vi "nanocal -- nuclear schottky fit V8.vi"() -> ()   [LabVIEW 2021] (continued)
\"στN\" -> 0.000000000000   ,  \"τ11 \" -> 0.000000000000   ,  \"τ12\" -> 0.000000000000   ,  \"τ22\" -> 0.000000000000   ,  \"τN1\" -> 0.000000000000   ,  \"τN2\" -> 0.000000000000   ,  \"σηlogτ1 \" -> 0.000000000000   ,  \"σηlogτS\" -> 0.000000000000   ,  \"σηlogτN\" -> 0.000000000000   ,  \"σlogτ1\" -> 0.000000000000   ,  \"σlogτS\" -> 0.000000000000   ,  \"σlogτN\" -> 0.000000000000   ,  \"σητ1\" -> 0.000000000000   ,  \"σητS \" -> 0.000000000000   ,  \"σητN\" -> 0.000000000000    |>   , \r\"IDS0648_220613_RAW_cal__ref_\" ->   <|    \"ζ\" -> 0.044166566928   ,  \"τ1\" -> 0.016574003526   ,  \"τS\" -> 0.032211448360   ,  \"τN\" -> 0.000936709307   ,  \"τC\" -> 0.001862438862   ,  \"κ0\" -> 0.000000003065   ,  \"mm1\" -> 0.000074801958   ,  \"mm2\" -> 0.015787727605   ,  \"mm3\" -> 0.037186110817   ,  \"T\" -> 0.520000000000   ,  \"B\" -> 6.000000000000   ,  \"θ\" -> 90.000000000000   ,  \"Reoff\" -> 0.000000000000   ,  \"Imoff\" -> 0.000000000000   ,  \"στ1\" -> 0.000113368552   ,  \"στS\" -> 0.000002764404   ,  \"στN\" -> 0.000003162403   ,  \"τ11 \" -> 0.000000000000   ,  \"τ12\" -> 0.000000000000   ,  \"τ22\" -> 0.000000000000   ,  \"τN1\" -> 0.000000000000   ,  \"τN2\" -> 0.000000000000   ,  \"σηlogτ1 \" -> 0.169044191232   ,  \"σηlogτS\" -> 0.000346748172   ,  \"σηlogτN\" -> 0.139725969375   ,  \"σlogτ1\" -> 0.006840142890   ,  \"σlogτS\" -> 0.000085820552   ,  \"σlogτN\" -> 0.003376077471   ,  \"σητ1\" -> 0.002801739022   ,  \"σητS \" -> 0.000011169261   ,  \"σητN\" -> 0.000130882616    |>   , \r\"IDS0648_220613_RAW_cal__sam_\" ->   <|    \"ζ\" -> 0.000000000000   ,  \"τ1\" -> 0.000000000000   ,  \"τS\" -> 0.000000000000   ,  \"τN\" -> 0.000000000000   ,  \"τC\" -> 0.000000000000   ,  \"κ0\" -> 0.000000000000   ,  \"mm1\" -> 0.000000000000   ,  \"mm2\" -> 0.000000000000   ,  \"mm3\" -> 0.000000000000   ,  \"T\" -> 0.520000000000   ,  \"B\" -> 6.000000000000   ,  \"θ\" -> 90.000000000000   ,  \"Reoff\" -> 0.000000000000   ,  \"Imoff\" -> 0.000000000000   ,  \"στ1\" -> 0.000000000000   ,  \"στS\" -> 0.000000000000   ,  \"στN\" -> 0.000000000000   ,  \"τ11 \" -> 0.000000000000   ,  \"τ12\" -> 0.000000000000   ,  \"τ22\" -> 0.000000000000   ,  \"τN1\" -> 0.000000000000   ,  \"τN2\" -> 0.000000000000   ,  \"σηlogτ1 \" -> 0.000000000000   ,  \"σηlogτS\" -> 0.000000000000   ,  \"σηlogτN\" -> 0.000000000000   ,  \"σlogτ1\" -> 0.000000000000   ,  \"σlogτS\" -> 0.000000000000   ,  \"σlogτN\" -> 0.000000000000   ,  \"σητ1\" -> 0.000000000000   ,  \"σητS \" -> 0.000000000000   ,  \"σητN\" -> 0.000000000000    |>   , \r\"IDS0649_220613_RAW_cal__ref_\" ->   <|    \"ζ\" -> 0.036098260006   ,  \"τ1\" -> 0.019839922246   ,  \"τS\" -> 0.028557133674   ,  \"τN\" -> 0.000530751010   ,  \"τC\" -> 0.002125743780   ,  \"κ0\" -> 0.000000003752   ,  \"mm1\" -> 0.000069248734   ,  \"mm2\" -> 0.019012462839   ,  \"mm3\" -> 0.033021861161   ,  \"T\" -> 0.620000000000   ,  \"B\" -> 6.000000000000   ,  \"θ\" -> 90.000000000000   ,  \"Reoff\" -> 0.000000000000   ,  \"Imoff\" -> 0.000000000000   ,  \"στ1\" -> 0.000292189890   ,  \"στS\" -> 0.000002960548   ,  \"στN\" -> 0.000003977957   ,  \"τ11 \" -> 0.000000000000   ,  \"τ12\" -> 0.000000000000   ,  \"τ22\" -> 0.000000000000   ,  \"τN1\" -> 0.000000000000   ,  \"τN2\" -> 0.000000000000   ,  \"σηlogτ1 \" -> 0.142367105799   ,  \"σηlogτS\" -> 0.000145255254   ,  \"σηlogτN\" -> 0.135095367098   ,  \"σlogτ1\" -> 0.014727370701   ,  \"σlogτS\" -> 0.000103671054   ,  \"σlogτN\" -> 0.007494959556   ,  \"σητ1\" -> 0.002824552309   ,  \"σητS \" -> 0.000004148074   ,  \"σητN\" -> 0.000071702003    |>   , \r\"IDS0649_220613_RAW_cal__sam_\" ->   <|    \"ζ\" -> 0.000000000000   ,  \"τ1\" -> 0.000000000000   ,  \"τS\" -> 0.000000000000   ,  \"τN\" -> 0.000000000000   ,  \"τC\" -> 0.000000000000   ,  \"κ0\" -> 0.000000000000   ,  \"mm1\" -> 0.000000000000   ,  \"mm2\" -> 0.000000000000   ,  \"mm3\" -> 0.000000000000   ,  \"T\" -> 0.620000000000   ,  \"B\" -> 6.000000000000   ,  \"θ\" -> 90.000000000000   ,  \"Reoff\" -> 0.000000000000   ,  \"Imoff\" -> 0.000000000000   ,  \"στ1\" -> 0.000000000000   ,  \"στS\" -> 0.000000000000   ,  \"στN\" -> 0.000000000000   ,  \"τ11 \" -> 0.000000000000   ,  \"τ12\" -> 0.000000000000   ,  \"τ22\" -> 0.000000000000   ,  \"τN1\" -> 0.000000000000   ,  \"τN2\" -> 0.000000000000   ,  \"σηlogτ1 \" -> 0.000000000000   ,  \"σηlogτS\" -> 0.000000000000   ,  \"σηlogτN\" -> 0.000000000000   ,  \"σlogτ1\" -> 0.000000000000   ,  \"σlogτS\" -> 0.000000000000   ,  \"σlogτN\" -> 0.000000000000   ,  \"σητ1\" -> 0.000000000000   ,  \"σητS \" -> 0.000000000000   ,  \"σητN\" -> 0.000000000000    |>   , \r\"IDS0650_220613_RAW_cal__ref_\" ->   <|    \"ζ\" -> 0.026767413186   ,  \"τ1\" -> 0.019958900137   ,  \"τS\" -> 0.023153953288   ,  \"τN\" -> 0.000189088054   ,  \"τC\" -> 0.002398350564   ,  \"κ0\" -> 0.000000005121   ,  \"mm1\" -> 0.000056918136   ,  \"mm2\" -> 0.019398352629   ,  \"mm3\" -> 0.026869854111   ,  \"T\" -> 0.820000000000   ,  \"B\" -> 6.000000000000   ,  \"θ\" -> 90.000000000000   ,  \"Reoff\" -> 0.000000000000   ,  \"Imoff\" -> 0.000000000000   ,  \"στ1\" -> 0.000637008577   ,  \"στS\" -> 0.000002061875   ,  \"στN\" -> 0.000003206406   ,  \"τ11 \" -> 0.000000000000   ,  \"τ12\" -> 0.000000000000   ,  \"τ22\" -> 0.000000000000   ,  \"τN1\" -> 0.000000000000   ,  \"τN2\" -> 0.000000000000   ,  \"σηlogτ1 \" -> 0.127380236705   ,  \"σηlogτS\" -> 0.000047088453   ,  \"σηlogτN\" -> 0.132172067620   ,  \"σlogτ1\" -> 0.031916016057   ,  \"σlogτS\" -> 0.000089050669   ,  \"σlogτN\" -> 0.016957208977   ,  \"σητ1\" -> 0.002542369424   ,  \"σητS \" -> 0.000001090284   ,  \"σητN\" -> 0.000024992159    |>   , \r\"IDS0650_220613_RAW_cal__sam_\" ->   <|    \"ζ\" -> 0.000000000000   ,  \"τ1\" -> 0.000000000000   ,  \"τS\" -> 0.000000000000   ,  \"τN\" -> 0.000000000000   ,  \"τC\" -> 0.000000000000   ,  \"κ0\" -> 0.000000000000   ,  \"mm1\" -> 0.000000000000   ,  \"mm2\" -> 0.000000000000   ,  \"mm3\" -> 0.000000000000   ,  \"T\" -> 0.820000000000   ,  \"B\" -> 6.000000000000   ,  \"θ\" -> 90.000000000000   ,  \"Reoff\" -> 0.000000000000   ,  \"Imoff\" -> 0.000000000000   ,  \"στ1\" -> 0.000000000000   ,  \"στS\" -> 0.000000000000   ,  \"στN\" -> 0.000000000000   ,  \"τ11 \" -> 0.000000000000   ,  \"τ12\" -> 0.000000000000   ,  \"τ22\" -> 0.000000000000   ,  \"τN1\" -> 0.000000000000   ,  \"τN2\" -> 0.000000000000   ,  \"σηlogτ1 \" -> 0.000000000000   ,  \"σηlogτS\" -> 0.000000000000   ,  \"σηlogτN\" -> 0.000000000000   ,  \"σlogτ1\" -> 0.000000000000   ,  \"σlogτS\" -> 0.000000000000   ,  \"σlogτN\" -> 0.000000000000   ,  \"σητ1\" -> 0.000000000000   ,  \"σητS \" -> 0.000000000000   ,  \"σητN\" -> 0.000000000000    |>   , \r\"IDS0651_220613_RAW_cal__ref_\" ->   <|    \"ζ\" -> 0.024620092111   ,  \"τ1\" -> 0.015537036119   ,  \"τS\" -> 0.019312906027   ,  \"τN\" -> 0.000067030104   ,  \"τC\" -> 0.002705916622   ,  \"κ0\" -> 0.000000007154   ,  \"mm1\" -> 0.000057343864   ,  \"mm2\" -> 0.015387205435   ,  \"mm3\" -> 0.022655475386   ,  \"T\" -> 1.120000000000   ,  \"B\" -> 6.000000000000   ,  \"θ\" -> 90.000000000000   ,  \"Reoff\" -> 0.000000000000   ,  \"Imoff\" -> 0.000000000000   ,  \"στ1\" -> 0.001880910040   ,  \"στS\" -> 0.000002935864   ,  \"στN\" -> 0.000004201788   ,  \"τ11 \" -> 0.000000000000   ,  \"τ12\" -> 0.000000000000   ,  \"τ22\" -> 0.000000000000   ,  \"τN1\" -> 0.000000000000   ,  \"τN2\" -> 0.000000000000   ,  \"σηlogτ1 \" -> 0.134633854477   ,  \"σηlogτS\" -> 0.000023496461   ,  \"σηlogτN\" -> 0.133516099454   ,  \"σlogτ1\" -> 0.121059771335   ,  \"σlogτS\" -> 0.000152015645   ,  \"σlogτN\" -> 0.062685083512   ,  \"σητ1\" -> 0.002091811060   ,  \"σητS \" -> 0.000000453785   ,  \"σητN\" -> 0.000008949598    |>   , \r\"IDS0651_220613_RAW_cal__sam_\" ->   <|    \"ζ\" -> 0.000000000000   ,  \"τ1\" -> 0.000000000000   ,  \"τS\" -> 0.000000000000   ,  \"τN\" -> 0.000000000000   ,  \"τC\" -> 0.000000000000   ,  \"κ0\" -> 0.000000000000   ,  \"mm1\" -> 0.000000000000   ,  \"mm2\" -> 0.000000000000   ,  \"mm3\" -> 0.000000000000   ,  \"T\" -> 1.120000000000   ,  \"B\" -> 6.000000000000   ,  \"θ\" -> 90.000000000000   ,  \"Reoff\" -> 0.000000000000   ,  \"Imoff\" -> 0.000000000000   ,  \"στ1\" -> 0.000000000000   ,  \"στS\" -> 0.000000000000   ,  \"στN\" -> 0.000000000000   ,  \"τ11 \" -> 0.000000000000   ,  \"τ12\" -> 0.000000000000   ,  \"τ22\" -> 0.000000000000   ,  \"τN1\" -> 0.000000000000   ,  \"τN2\" -> 0.000000000000   ,  \"σηlogτ1 \" -> 0.000000000000   ,  \"σηlogτS\" -> 0.000000000000   ,  \"σηlogτN\" -> 0.000000000000   ,  \"σlogτ1\" -> 0.000000000000   ,  \"σlogτS\" -> 0.000000000000   ,  \"σlogτN\" -> 0.000000000000   ,  \"σητ1\" -> 0.000000000000   ,  \"σητS \" -> 0.000000000000   ,  \"σητN\" -> 0.000000000000    |>   , \r\"IDS0652_220613_RAW_cal__ref_\" ->   <|    \"ζ\" -> 0.018133168210   ,  \"τ1\" -> 0.015564889407   ,  \"τS\" -> 0.014281099211   ,  \"τN\" -> 0.000013869214   ,  \"τC\" -> 0.003052925154   ,  \"κ0\" -> 0.000000012545   ,  \"mm1\" -> 0.000045053166   ,  \"mm2\" -> 0.015460375194   ,  \"mm3\" -> 0.017666567693   ,  \"T\" -> 1.900000000000   ,  \"B\" -> 6.000000000000   ,  \"θ\" -> 90.000000000000   ,  \"Reoff\" -> 0.000000000000   ,  \"Imoff\" -> 0.000000000000   ,  \"στ1\" -> 0.007531531497   ,  \"στS\" -> 0.000002103829   ,  \"στN\" -> 0.000003717358   ,  \"τ11 \" -> 0.000000000000   ,  \"τ12\" -> 0.000000000000   ,  \"τ22\" -> 0.000000000000   ,  \"τN1\" -> 0.000000000000   ,  \"τN2\" -> 0.000000000000   ,  \"σηlogτ1 \" -> 0.117619771927   ,  \"σηlogτS\" -> 0.000004424081   ,  \"σηlogτN\" -> 0.130136475948   ,  \"σlogτ1\" -> 0.483879538125   ,  \"σlogτS\" -> 0.000147315653   ,  \"σlogτN\" -> 0.268029442413   ,  \"σητ1\" -> 0.001830738742   ,  \"σητS \" -> 0.000000063181   ,  \"σητN\" -> 0.000001804891    |>   , \r\"IDS0652_220613_RAW_cal__sam_\" ->   <|    \"ζ\" -> 0.000000000000   ,  \"τ1\" -> 0.000000000000   ,  \"τS\" -> 0.000000000000   ,  \"τN\" -> 0.000000000000   ,  \"τC\" -> 0.000000000000   ,  \"κ0\" -> 0.000000000000   ,  \"mm1\" -> 0.000000000000   ,  \"mm2\" -> 0.000000000000   ,  \"mm3\" -> 0.000000000000   ,  \"T\" -> 1.900000000000   ,  \"B\" -> 6.000000000000   ,  \"θ\" -> 90.000000000000   ,  \"Reoff\" -> 0.000000000000   ,  \"Imoff\" -> 0.000000000000   ,  \"στ1\" -> 0.000000000000   ,  \"στS\" -> 0.000000000000   ,  \"στN\" -> 0.000000000000   ,  \"τ11 \" -> 0.000000000000   ,  \"τ12\" -> 0.000000000000   ,  \"τ22\" -> 0.000000000000   ,  \"τN1\" -> 0.000000000000   ,  \"τN2\" -> 0.000000000000   ,  \"σηlogτ1 \" -> 0.000000000000   ,  \"σηlogτS\" -> 0.000000000000   ,  \"σηlogτN\" -> 0.000000000000   ,  \"σlogτ1\" -> 0.000000000000   ,  \"σlogτS\" -> 0.000000000000   ,  \"σlogτN\" -> 0.000000000000   ,  \"σητ1\" -> 0.000000000000   ,  \"σητS \" -> 0.000000000000   ,  \"σητN\" -> 0.000000000000    |>   , \r\"IDS0653_220613_RAW_cal__ref_\" ->   <|    \"ζ\" -> 0.015908509188   ,  \"τ1\" -> 0.015560123784   ,  \"τS\" -> 0.010437245612   ,  \"τN\" -> 0.000002583564   ,  \"τC\" -> 0.002705916622   ,  \"κ0\" -> 0.000000022391   ,  \"mm1\" -> 0.000033844139   ,  \"mm2\" -> 0.013260236096   ,  \"mm3\" -> 0.015577871465   ,  \"T\" -> 3.100000000000   ,  \"B\" -> 6.000000000000   ,  \"θ\" -> 90.000000000000   ,  \"Reoff\" -> 0.000000000000   ,  \"Imoff\" -> 0.000000000000   ,  \"στ1\" -> 0.028222346539   ,  \"στS\" -> 0.000001217229   ,  \"στN\" -> 0.000002849695   ,  \"τ11 \" -> 0.000000000000   ,  \"τ12\" -> 0.000000000000   ,  \"τ22\" -> 0.000000000000   ,  \"τN1\" -> 0.000000000000   ,  \"τN2\" -> 0.000000000000   ,  \"σηlogτ1 \" -> 0.102372166935   ,  \"σηlogτS\" -> 0.000000706034   ,  \"σηlogτN\" -> 0.126762129997   ,  \"σlogτ1\" -> 1.813761055527   ,  \"σlogτS\" -> 0.000116623590   ,  \"σlogτN\" -> 1.103009360706   ,  \"σητ1\" -> 0.001592923590   ,  \"σητS \" -> 0.000000007369   ,  \"σητN\" -> 0.000000327498    |>   , \r\"IDS0653_220613_RAW_cal__sam_\" ->   <|    \"ζ\" -> 0.000000000000   ,  \"τ1\" -> 0.000000000000   ,  \"τS\" -> 0.000000000000   ,  \"τN\" -> 0.000000000000   ,  \"τC\" -> 0.000000000000   ,  \"κ0\" -> 0.000000000000   ,  \"mm1\" -> 0.000000000000   ,  \"mm2\" -> 0.000000000000   ,  \"mm3\" -> 0.000000000000   ,  \"T\" -> 3.100000000000   ,  \"B\" -> 6.000000000000   ,  \"θ\" -> 90.000000000000   ,  \"Reoff\" -> 0.000000000000   ,  \"Imoff\" -> 0.000000000000   ,  \"στ1\" -> 0.000000000000   ,  \"στS\" -> 0.000000000000   ,  \"στN\" -> 0.000000000000   ,  \"τ11 \" -> 0.000000000000   ,  \"τ12\" -> 0.000000000000   ,  \"τ22\" -> 0.000000000000   ,  \"τN1\" -> 0.000000000000   ,  \"τN2\" -> 0.000000000000   ,  \"σηlogτ1 \" -> 0.000000000000   ,  \"σηlogτS\" -> 0.000000000000   ,  \"σηlogτN\" -> 0.000000000000   ,  \"σlogτ1\" -> 0.000000000000   ,  \"σlogτS\" -> 0.000000000000   ,  \"σlogτN\" -> 0.000000000000   ,  \"σητ1\" -> 0.000000000000   ,  \"σητS \" -> 0.000000000000   ,  \"σητN\" -> 0.000000000000    |>   , \r\"IDS0654_220613_RAW_cal__ref_\" ->   <|    \"ζ\" -> 0.019038104176   ,  \"τ1\" -> 0.015490030186   ,  \"τS\" -> 0.006638290269   ,  \"τN\" -> 0.000000433283   ,  \"τC\" -> 0.001884122649   ,  \"κ0\" -> 0.000000055099   ,  \"mm1\" -> 0.000027619939   ,  \"mm2\" -> 0.008620619838   ,  \"mm3\" -> 0.015491025321   ,  \"T\" -> 5.700000000000   ,  \"B\" -> 6.000000000000   ,  \"θ\" -> 90.000000000000   ,  \"Reoff\" -> 0.000000000000   ,  \"Imoff\" -> 0.000000000000   ,  \"στ1\" -> 0.134458541237   ,  \"στS\" -> 0.000000694139   ,  \"στN\" -> 0.000002640501   ,  \"τ11 \" -> 0.000000000000   ,  \"τ12\" -> 0.000000000000   ,  \"τ22\" -> 0.000000000000   ,  \"τN1\" -> 0.000000000000   ,  \"τN2\" -> 0.000000000000   ,  \"σηlogτ1 \" -> 0.085447105740   ,  \"σηlogτS\" -> 0.000000087953   ,  \"σηlogτN\" -> 0.122534708662   ,  \"σlogτ1\" -> 8.680327902656   ,  \"σlogτS\" -> 0.000104565901   ,  \"σlogτN\" -> 6.094171441911   ,  \"σητ1\" -> 0.001323578247   ,  \"σητS \" -> 0.000000000584   ,  \"σητN\" -> 0.000000053092    |>   , \r\"IDS0654_220613_RAW_cal__sam_\" ->   <|    \"ζ\" -> 0.000000000000   ,  \"τ1\" -> 0.000000000000   ,  \"τS\" -> 0.000000000000   ,  \"τN\" -> 0.000000000000   ,  \"τC\" -> 0.000000000000   ,  \"κ0\" -> 0.000000000000   ,  \"mm1\" -> 0.000000000000   ,  \"mm2\" -> 0.000000000000   ,  \"mm3\" -> 0.000000000000   ,  \"T\" -> 5.700000000000   ,  \"B\" -> 6.000000000000   ,  \"θ\" -> 90.000000000000   ,  \"Reoff\" -> 0.000000000000   ,  \"Imoff\" -> 0.000000000000   ,  \"στ1\" -> 0.000000000000   ,  \"στS\" -> 0.000000000000   ,  \"στN\" -> 0.000000000000   ,  \"τ11 \" -> 0.000000000000   ,  \"τ12\" -> 0.000000000000   ,  \"τ22\" -> 0.000000000000   ,  \"τN1\" -> 0.000000000000   ,  \"τN2\" -> 0.000000000000   ,  \"σηlogτ1 \" -> 0.000000000000   ,  \"σηlogτS\" -> 0.000000000000   ,  \"σηlogτN\" -> 0.000000000000   ,  \"σlogτ1\" -> 0.000000000000   ,  \"σlogτS\" -> 0.000000000000   ,  \"σlogτN\" -> 0.000000000000   ,  \"σητ1\" -> 0.000000000000   ,  \"σητS \" -> 0.000000000000   ,  \"σητN\" -> 0.000000000000    |>   , \r\"IDS0656_220614_RAW_cal__ref_\" ->   <|    \"ζ\" -> 0.110263031005   ,  \"τ1\" -> 0.036264946317   ,  \"τS\" -> 0.035363841561   ,  \"τN\" -> 0.002907549875   ,  \"τC\" -> 0.001147321567   ,  \"κ0\" -> 0.000000001565   ,  \"mm1\" -> 0.000111012610   ,  \"mm2\" -> 0.028483762527   ,  \"mm3\" -> 0.051308803803   ,  \"T\" -> 0.300000000000   ,  \"B\" -> 4.000000000000   ,  \"θ\" -> 90.000000000000   ,  \"Reoff\" -> 0.000000000000   ,  \"Imoff\" -> 0.000000000000   ,  \"στ1\" -> 0.000283051813   ,  \"στS\" -> 0.000006866298   ,  \"στN\" -> 0.000012798500   ,  \"τ11 \" -> 0.000000000000   ,  \"τ12\" -> 0.000000000000   ,  \"τ22\" -> 0.000000000000   ,  \"τN1\" -> 0.000000000000   ,  \"τN2\" -> 0.000000000000   ,  \"σηlogτ1 \" -> 0.116599052310   ,  \"σηlogτS\" -> 0.000355346389   ,  \"σηlogτN\" -> 0.130406494845   ,  \"σlogτ1\" -> 0.007805107735   ,  \"σlogτS\" -> 0.000194161553   ,  \"σlogτN\" -> 0.004401816116   ,  \"σητ1\" -> 0.004228458373   ,  \"σητS \" -> 0.000012566413   ,  \"σητN\" -> 0.000379163388    |>   , \r\"IDS0656_220614_RAW_cal__sam_\" ->   <|    \"ζ\" -> 0.000000000000   ,  \"τ1\" -> 0.000000000000   ,  \"τS\" -> 0.000000000000   ,  \"τN\" -> 0.000000000000   ,  \"τC\" -> 0.000000000000   ,  \"κ0\" -> 0.000000000000   ,  \"mm1\" -> 0.000000000000   ,  \"mm2\" -> 0.000000000000   ,  \"mm3\" -> 0.000000000000   ,  \"T\" -> 0.300000000000   ,  \"B\" -> 4.000000000000   ,  \"θ\" -> 90.000000000000   ,  \"Reoff\" -> 0.000000000000   ,  \"Imoff\" -> 0.000000000000   ,  \"στ1\" -> 0.000000000000   ,  \"στS\" -> 0.000000000000   ,  \"στN\" -> 0.000000000000   ,  \"τ11 \" -> 0.000000000000   ,  \"τ12\" -> 0.000000000000   ,  \"τ22\" -> 0.000000000000   ,  \"τN1\" -> 0.000000000000   ,  \"τN2\" -> 0.000000000000   ,  \"σηlogτ1 \" -> 0.000000000000   ,  \"σηlogτS\" -> 0.000000000000   ,  \"σηlogτN\" -> 0.000000000000   ,  \"σlogτ1\" -> 0.000000000000   ,  \"σlogτS\" -> 0.000000000000   ,  \"σlogτN\" -> 0.000000000000   ,  \"σητ1\" -> 0.000000000000   ,  \"σητS \" -> 0.000000000000   ,  \"σητN\" -> 0.000000000000    |>   , \r"
  in  "string IN":string="  \"IDS0158_210310_RAW_cal__ref_\" ->   <|    \"ζ\" -> 0.342934102355   ,  \"τ1\" -> 0.037912336866   ,  \"τS\" -> 0.322770587290   ,  \"τN\" -> 0.224517468406   ,  \"τC\" -> 0.000970428995   ,  \"κ0\" -> 0.000000000517   ,  \"mm1\" -> 0.000247395955   ,  \"mm2\" -> 0.021898106728   ,  \"mm3\" -> 0.751709056984   ,  \"T\" -> 0.120000000000   ,  \"B\" -> 12.000000000000   ,  \"θ\" -> 0.000000000000   ,  \"Reoff\" -> 0.000000000000   ,  \"Imoff\" -> 0.000000000000   ,  \"στ1\" -> 0.000893425914   ,  \"στS\" -> 0.002489408176   ,  \"στN\" -> 0.002611842121   ,  \"τ11 \" -> 0.000000000000   ,  \"τ12\" -> 0.000000000000   ,  \"τ22\" -> 0.000000000000   ,  \"τN1\" -> 0.000000000000   ,  \"τN2\" -> 0.000000000000   ,  \"σηlogτ1 \" -> 0.114569772809   ,  \"σηlogτS\" -> 0.007573309274   ,  \"σηlogτN\" -> 0.068166495911   ,  \"σlogτ1\" -> 0.023565572257   ,  \"σlogτS\" -> 0.007712623993   ,  \"σlogτN\" -> 0.011633135451   ,  \"σητ1\" -> 0.004343607821   ,  \"σητS \" -> 0.002444441482   ,  \"σητN\" -> 0.015304569092    |>   , \n\"IDS0158_210310_RAW_cal__sam_\" ->   <|    \"ζ\" -> 0.286336668596   ,  \"τ1\" -> 0.037477267671   ,  \"τS\" -> 0.354459287884   ,  \"τN\" -> 0.444916383639   ,  \"τC\" -> 0.001225600579   ,  \"κ0\" -> 0.000000000596   ,  \"mm1\" -> 0.000272242393   ,  \"mm2\" -> 0.016302418461   ,  \"mm3\" -> 1.050394445660   ,  \"T\" -> 0.120000000000   ,  \"B\" -> 12.000000000000   ,  \"θ\" -> 0.000000000000   ,  \"Reoff\" -> 0.000000000000   ,  \"Imoff\" -> 0.000000000000   ,  \"στ1\" -> 0.000000000000   ,  \"στS\" -> 0.000000000000   ,  \"στN\" -> 0.000000000000   ,  \"τ11 \" -> 0.000000000000   ,  \"τ12\" -> 0.000000000000   ,  \"τ22\" -> 0.000000000000   ,  \"τN1\" -> 0.000000000000   ,  \"τN2\" -> 0.000000000000   ,  \"σηlogτ1 \" -> 0.000000000000   ,  \"σηlogτS\" -> 0.000000000000   ,  \"σηlogτN\" -> 0.000000000000   ,  \"σlogτ1\" -> 0.000000000000   ,  \"σlogτS\" -> 0.000000000000   ,  \"σlogτN\" -> 0.000000000000   ,  \"σητ1\" -> 0.000000000000   ,  \"σητS \" -> 0.000000000000   ,  \"σητN\" -> 0.000000000000    |>   , \n\"IDS0159_210310_RAW_cal__ref_\" ->   <|    \"ζ\" -> 0.271761862806   ,  \"τ1\" -> 0.039955104592   ,  \"τS\" -> 0.227503722031   ,  \"τN\" -> 0.142080712192   ,  \"τC\" -> 0.000995450305   ,  \"κ0\" -> 0.000000000652   ,  \"mm1\" -> 0.000212140795   ,  \"mm2\" -> 0.023804196565   ,  \"mm3\" -> 0.486957606069   ,  \"T\" -> 0.150000000000   ,  \"B\" -> 12.000000000000   ,  \"θ\" -> 0.000000000000   ,  \"Reoff\" -> 0.000000000000   ,  \"Imoff\" -> 0.000000000000   ,  \"στ1\" -> 0.000698593116   ,  \"στS\" -> 0.001142949493   ,  \"στN\" -> 0.001230291496   ,  \"τ11 \" -> 0.000000000000   ,  \"τ12\" -> 0.000000000000   ,  \"τ22\" -> 0.000000000000   ,  \"τN1\" -> 0.000000000000   ,  \"τN2\" -> 0.000000000000   ,  \"σηlogτ1 \" -> 0.100498796621   ,  \"σηlogτS\" -> 0.005660617730   ,  \"σηlogτN\" -> 0.063140982058   ,  \"σlogτ1\" -> 0.017484452181   ,  \"σlogτS\" -> 0.005023871622   ,  \"σlogτN\" -> 0.008659102821   ,  \"σητ1\" -> 0.004015439930   ,  \"σητS \" -> 0.001287811603   ,  \"σητN\" -> 0.008971115699    |>   , \n\"IDS0159_210310_RAW_cal__sam_\" ->   <|    \"ζ\" -> 0.219100303741   ,  \"τ1\" -> 0.028643012604   ,  \"τS\" -> 0.279362928811   ,  \"τN\" -> 0.246156444058   ,  \"τC\" -> 0.001272401549   ,  \"κ0\" -> 0.000000000760   ,  \"mm1\" -> 0.000227975653   ,  \"mm2\" -> 0.014929571562   ,  \"mm3\" -> 0.655418694024   ,  \"T\" -> 0.150000000000   ,  \"B\" -> 12.000000000000   ,  \"θ\" -> 0.000000000000   ,  \"Reoff\" -> 0.000000000000   ,  \"Imoff\" -> 0.000000000000   ,  \"στ1\" -> 0.000000000000   ,  \"στS\" -> 0.000000000000   ,  \"στN\" -> 0.000000000000   ,  \"τ11 \" -> 0.000000000000   ,  \"τ12\" -> 0.000000000000   ,  \"τ22\" -> 0.000000000000   ,  \"τN1\" -> 0.000000000000   ,  \"τN2\" -> 0.000000000000   ,  \"σηlogτ1 \" -> 0.000000000000   ,  \"σηlogτS\" -> 0.000000000000   ,  \"σηlogτN\" -> 0.000000000000   ,  \"σlogτ1\" -> 0.000000000000   ,  \"σlogτS\" -> 0.000000000000   ,  \"σlogτN\" -> 0.000000000000   ,  \"σητ1\" -> 0.000000000000   ,  \"σητS \" -> 0.000000000000   ,  \"σητN\" -> 0.000000000000    |>   , \n\"IDS0160_210310_RAW_cal__ref_\" ->   <|    \"ζ\" -> 0.199613086212   ,  \"τ1\" -> 0.022193731398   ,  \"τS\" -> 0.116862561742   ,  \"τN\" -> 0.097247059130   ,  \"τC\" -> 0.001045881960   ,  \"κ0\" -> 0.000000000931   ,  \"mm1\" -> 0.000172948552   ,  \"mm2\" -> 0.011671612475   ,  \"mm3\" -> 0.268243755414   ,  \"T\" -> 0.180000000000   ,  \"B\" -> 12.000000000000   ,  \"θ\" -> 0.000000000000   ,  \"Reoff\" -> 0.000000000000   ,  \"Imoff\" -> 0.000000000000   ,  \"στ1\" -> 0.000089856815   ,  \"στS\" -> 0.000165029214   ,  \"στN\" -> 0.000188286128   ,  \"τ11 \" -> 0.000000000000   ,  \"τ12\" -> 0.000000000000   ,  \"τ22\" -> 0.000000000000   ,  \"τN1\" -> 0.000000000000   ,  \"τN2\" -> 0.000000000000   ,  \"σηlogτ1 \" -> 0.093550953866   ,  \"σηlogτS\" -> 0.006075230131   ,  \"σηlogτN\" -> 0.064015363974   ,  \"σlogτ1\" -> 0.004048747519   ,  \"σlogτS\" -> 0.001412164955   ,  \"σlogτN\" -> 0.001936162698   ,  \"σητ1\" -> 0.002076244742   ,  \"σητS \" -> 0.000709966956   ,  \"σητN\" -> 0.006225305886    |>   , \n\"IDS0160_210310_RAW_cal__sam_\" ->   <|    \"ζ\" -> 0.170488637524   ,  \"τ1\" -> 0.029234231120   ,  \"τS\" -> 0.149095458227   ,  \"τN\" -> 0.151792620275   ,  \"τC\" -> 0.001113424175   ,  \"κ0\" -> 0.000000001042   ,  \"mm1\" -> 0.000161291869   ,  \"mm2\" -> 0.013922632736   ,  \"mm3\" -> 0.368449807743   ,  \"T\" -> 0.180000000000   ,  \"B\" -> 12.000000000000   ,  \"θ\" -> 0.000000000000   ,  \"Reoff\" -> 0.000000000000   ,  \"Imoff\" -> 0.000000000000   ,  \"στ1\" -> 0.000000000000   ,  \"στS\" -> 0.000000000000   ,  \"στN\" -> 0.000000000000   ,  \"τ11 \" -> 0.000000000000   ,  \"τ12\" -> 0.000000000000   ,  \"τ22\" -> 0.000000000000   ,  \"τN1\" -> 0.000000000000   ,  \"τN2\" -> 0.000000000000   ,  \"σηlogτ1 \" -> 0.000000000000   ,  \"σηlogτS\" -> 0.000000000000   ,  \"σηlogτN\" -> 0.000000000000   ,  \"σlogτ1\" -> 0.000000000000   ,  \"σlogτS\" -> 0.000000000000   ,  \"σlogτN\" -> 0.000000000000   ,  \"σητ1\" -> 0.000000000000   ,  \"σητS \" -> 0.000000000000   ,  \"σητN\" -> 0.000000000000    |>   , \n\"IDS0161_210310_RAW_cal__ref_\" ->   <|    \"ζ\" -> 0.155485326727   ,  \"τ1\" -> 0.024589160211   ,  \"τS\" -> 0.103187251839   ,  \"τN\" -> 0.059327264902   ,  \"τC\" -> 0.001362397594   ,  \"κ0\" -> 0.000000001075   ,  \"mm1\" -> 0.000181522487   ,  \"mm2\" -> 0.014905594718   ,  \"mm3\" -> 0.198647580074   ,  \"T\" -> 0.200000000000   ,  \"B\" -> 12.000000000000   ,  \"θ\" -> 0.000000000000   ,  \"Reoff\" -> 0.000000000000   ,  \"Imoff\" -> 0.000000000000   ,  \"στ1\" -> 0.000106824093   ,  \"στS\" -> 0.000114207069   ,  \"στN\" -> 0.000127738509   ,  \"τ11 \" -> 0.000000000000   ,  \"τ12\" -> 0.000000000000   ,  \"τ22\" -> 0.000000000000   ,  \"τN1\" -> 0.000000000000   ,  \"τN2\" -> 0.000000000000   ,  \"σηlogτ1 \" -> 0.086294510505   ,  \"σηlogτS\" -> 0.004144737065   ,  \"σηlogτN\" -> 0.058529518145   ,  \"σlogτ1\" -> 0.004344357106   ,  \"σlogτS\" -> 0.001106794371   ,  \"σlogτN\" -> 0.002153116435   ,  \"σητ1\" -> 0.002121909544   ,  \"σητS \" -> 0.000427684027   ,  \"σητN\" -> 0.003472396228    |>   , \n\"IDS0161_210310_RAW_cal__sam_\" ->   <|    \"ζ\" -> 0.130531197151   ,  \"τ1\" -> 0.025704482770   ,  \"τS\" -> 0.129606657196   ,  \"τN\" -> 0.091602369165   ,  \"τC\" -> 0.001441379995   ,  \"κ0\" -> 0.000000001211   ,  \"mm1\" -> 0.000164978070   ,  \"mm2\" -> 0.014468182937   ,  \"mm3\" -> 0.262596407151   ,  \"T\" -> 0.200000000000   ,  \"B\" -> 12.000000000000   ,  \"θ\" -> 0.000000000000   ,  \"Reoff\" -> 0.000000000000   ,  \"Imoff\" -> 0.000000000000   ,  \"στ1\" -> 0.000000000000   ,  \"στS\" -> 0.000000000000   ,  \"στN\" -> 0.000000000000   ,  \"τ11 \" -> 0.000000000000   ,  \"τ12\" -> 0.000000000000   ,  \"τ22\" -> 0.000000000000   ,  \"τN1\" -> 0.000000000000   ,  \"τN2\" -> 0.000000000000   ,  \"σηlogτ1 \" -> 0.000000000000   ,  \"σηlogτS\" -> 0.000000000000   ,  \"σηlogτN\" -> 0.000000000000   ,  \"σlogτ1\" -> 0.000000000000   ,  \"σlogτS\" -> 0.000000000000   ,  \"σlogτN\" -> 0.000000000000   ,  \"σητ1\" -> 0.000000000000   ,  \"σητS \" -> 0.000000000000   ,  \"σητN\" -> 0.000000000000    |>   , \n\"IDS0162_210310_RAW_cal__ref_\" ->   <|    \"ζ\" -> 0.085932974943   ,  \"τ1\" -> 0.018822470857   ,  \"τS\" -> 0.068810147904   ,  \"τN\" -> 0.024216831887   ,  \"τC\" -> 0.001953952621   ,  \"κ0\" -> 0.000000001388   ,  \"mm1\" -> 0.000150968751   ,  \"mm2\" -> 0.013294741414   ,  \"mm3\" -> 0.108351778227   ,  \"T\" -> 0.250000000000   ,  \"B\" -> 12.000000000000   ,  \"θ\" -> 0.000000000000   ,  \"Reoff\" -> 0.000000000000   ,  \"Imoff\" -> 0.000000000000   ,  \"στ1\" -> 0.000058321163   ,  \"στS\" -> 0.000035049706   ,  \"στN\" -> 0.000037861271   ,  \"τ11 \" -> 0.000000000000   ,  \"τ12\" -> 0.000000000000   ,  \"τ22\" -> 0.000000000000   ,  \"τN1\" -> 0.000000000000   ,  \"τN2\" -> 0.000000000000   ,  \"σηlogτ1 \" -> 0.080513059924   ,  \"σηlogτS\" -> 0.002518022810   ,  \"σηlogτN\" -> 0.054257654253   ,  \"σlogτ1\" -> 0.003098486056   ,  \"σlogτS\" -> 0.000509368271   ,  \"σlogτN\" -> 0.001563427918   ,  \"σητ1\" -> 0.001515454724   ,  \"σητS \" -> 0.000173265522   ,  \"σητN\" -> 0.001313948492    |>   , \n\"IDS0162_210310_RAW_cal__sam_\" ->   <|    \"ζ\" -> 0.078258046754   ,  \"τ1\" -> 0.028009840731   ,  \"τS\" -> 0.092122038762   ,  \"τN\" -> 0.030129595899   ,  \"τC\" -> 0.001641062244   ,  \"κ0\" -> 0.000000001543   ,  \"mm1\" -> 0.000117303440   ,  \"mm2\" -> 0.019983073008   ,  \"mm3\" -> 0.141369335330   ,  \"T\" -> 0.250000000000   ,  \"B\" -> 12.000000000000   ,  \"θ\" -> 0.000000000000   ,  \"Reoff\" -> 0.000000000000   ,  \"Imoff\" -> 0.000000000000   ,  \"στ1\" -> 0.000000000000   ,  \"στS\" -> 0.000000000000   ,  \"στN\" -> 0.000000000000   ,  \"τ11 \" -> 0.000000000000   ,  \"τ12\" -> 0.000000000000   ,  \"τ22\" -> 0.000000000000   ,  \"τN1\" -> 0.000000000000   ,  \"τN2\" -> 0.000000000000   ,  \"σηlogτ1 \" -> 0.000000000000   ,  \"σηlogτS\" -> 0.000000000000   ,  \"σηlogτN\" -> 0.000000000000   ,  \"σlogτ1\" -> 0.000000000000   ,  \"σlogτS\" -> 0.000000000000   ,  \"σlogτN\" -> 0.000000000000   ,  \"σητ1\" -> 0.000000000000   ,  \"σητS \" -> 0.000000000000   ,  \"σητN\" -> 0.000000000000    |>   , \n\"IDS0163_210310_RAW_cal__ref_\" ->   <|    \"ζ\" -> 0.058825748663   ,  \"τ1\" -> 0.015012107932   ,  \"τS\" -> 0.052128918860   ,  \"τN\" -> 0.012953217864   ,  \"τC\" -> 0.002393557537   ,  \"κ0\" -> 0.000000001766   ,  \"mm1\" -> 0.000127725677   ,  \"mm2\" -> 0.011559700576   ,  \"mm3\" -> 0.074628881357   ,  \"T\" -> 0.300000000000   ,  \"B\" -> 12.000000000000   ,  \"θ\" -> 0.000000000000   ,  \"Reoff\" -> 0.000000000000   ,  \"Imoff\" -> 0.000000000000   ,  \"στ1\" -> 0.000023064935   ,  \"στS\" -> 0.000009573131   ,  \"στN\" -> 0.000010092664   ,  \"τ11 \" -> 0.000000000000   ,  \"τ12\" -> 0.000000000000   ,  \"τ22\" -> 0.000000000000   ,  \"τN1\" -> 0.000000000000   ,  \"τN2\" -> 0.000000000000   ,  \"σηlogτ1 \" -> 0.078709092172   ,  \"σηlogτS\" -> 0.001802886041   ,  \"σηlogτN\" -> 0.052574057148   ,  \"σlogτ1\" -> 0.001536422126   ,  \"σlogτS\" -> 0.000183643382   ,  \"σlogτN\" -> 0.000779162669   ,  \"σητ1\" -> 0.001181589387   ,  \"σητS \" -> 0.000093982500   ,  \"σητN\" -> 0.000681003216    |>   , \n\"IDS0163_210310_RAW_cal__sam_\" ->   <|    \"ζ\" -> 0.054088186012   ,  \"τ1\" -> 0.023838802615   ,  \"τS\" -> 0.069079396629   ,  \"τN\" -> 0.016435267456   ,  \"τC\" -> 0.002025071743   ,  \"κ0\" -> 0.000000001955   ,  \"mm1\" -> 0.000101234646   ,  \"mm2\" -> 0.018244822177   ,  \"mm3\" -> 0.097657814678   ,  \"T\" -> 0.300000000000   ,  \"B\" -> 12.000000000000   ,  \"θ\" -> 0.000000000000   ,  \"Reoff\" -> 0.000000000000   ,  \"Imoff\" -> 0.000000000000   ,  \"στ1\" -> 0.000000000000   ,  \"στS\" -> 0.000000000000   ,  \"στN\" -> 0.000000000000   ,  \"τ11 \" -> 0.000000000000   ,  \"τ12\" -> 0.000000000000   ,  \"τ22\" -> 0.000000000000   ,  \"τN1\" -> 0.000000000000   ,  \"τN2\" -> 0.000000000000   ,  \"σηlogτ1 \" -> 0.000000000000   ,  \"σηlogτS\" -> 0.000000000000   ,  \"σηlogτN\" -> 0.000000000000   ,  \"σlogτ1\" -> 0.000000000000   ,  \"σlogτS\" -> 0.000000000000   ,  \"σlogτN\" -> 0.000000000000   ,  \"σητ1\" -> 0.000000000000   ,  \"σητS \" -> 0.000000000000   ,  \"σητN\" -> 0.000000000000    |>   , \n\"IDS0164_210310_RAW_cal__ref_\" ->   <|    \"ζ\" -> 0.042805749253   ,  \"τ1\" -> 0.013206199214   ,  \"τS\" -> 0.042245691100   ,  \"τN\" -> 0.007144228501   ,  \"τC\" -> 0.002899499229   ,  \"κ0\" -> 0.000000002181   ,  \"mm1\" -> 0.000111927858   ,  \"mm2\" -> 0.010938028304   ,  \"mm3\" -> 0.056559834396   ,  \"T\" -> 0.360000000000   ,  \"B\" -> 12.000000000000   ,  \"θ\" -> 0.000000000000   ,  \"Reoff\" -> 0.000000000000   ,  \"Imoff\" -> 0.000000000000   ,  \"στ1\" -> 0.000012292384   ,  \"στS\" -> 0.000003241338   ,  \"στN\" -> 0.000003368378   ,  \"τ11 \" -> 0.000000000000   ,  \"τ12\" -> 0.000000000000   ,  \"τ22\" -> 0.000000000000   ,  \"τN1\" -> 0.000000000000   ,  \"τN2\" -> 0.000000000000   ,  \"σηlogτ1 \" -> 0.075974060792   ,  \"σηlogτS\" -> 0.001194926073   ,  \"σηlogτN\" -> 0.051138297484   ,  \"σlogτ1\" -> 0.000930804037   ,  \"σlogτS\" -> 0.000076725884   ,  \"σlogτN\" -> 0.000471482447   ,  \"σητ1\" -> 0.001003328582   ,  \"σητS \" -> 0.000050480478   ,  \"σητN\" -> 0.000365343682    |>   , \n\"IDS0164_210310_RAW_cal__sam_\" ->   <|    \"ζ\" -> 0.039314966212   ,  \"τ1\" -> 0.020712803909   ,  \"τS\" -> 0.055413767550   ,  \"τN\" -> 0.008474403424   ,  \"τC\" -> 0.002674063387   ,  \"κ0\" -> 0.000000002415   ,  \"mm1\" -> 0.000096818147   ,  \"mm2\" -> 0.017190811405   ,  \"mm3\" -> 0.072499170001   ,  \"T\" -> 0.360000000000   ,  \"B\" -> 12.000000000000   ,  \"θ\" -> 0.000000000000   ,  \"Reoff\" -> 0.000000000000   ,  \"Imoff\" -> 0.000000000000   ,  \"στ1\" -> 0.000000000000   ,  \"στS\" -> 0.000000000000   ,  \"στN\" -> 0.000000000000   ,  \"τ11 \" -> 0.000000000000   ,  \"τ12\" -> 0.000000000000   ,  \"τ22\" -> 0.000000000000   ,  \"τN1\" -> 0.000000000000   ,  \"τN2\" -> 0.000000000000   ,  \"σηlogτ1 \" -> 0.000000000000   ,  \"σηlogτS\" -> 0.000000000000   ,  \"σηlogτN\" -> 0.000000000000   ,  \"σlogτ1\" -> 0.000000000000   ,  \"σlogτS\" -> 0.000000000000   ,  \"σlogτN\" -> 0.000000000000   ,  \"σητ1\" -> 0.000000000000   ,  \"σητS \" -> 0.000000000000   ,  \"σητN\" -> 0.000000000000    |>   , \n\"IDS0165_210310_RAW_cal__ref_\" ->   <|    \"ζ\" -> 0.032274621211   ,  \"τ1\" -> 0.011425652621   ,  \"τS\" -> 0.034817148793   ,  \"τN\" -> 0.004293407669   ,  \"τC\" -> 0.003209213512   ,  \"κ0\" -> 0.000000002697   ,  \"mm1\" -> 0.000092323212   ,  \"mm2\" -> 0.009918344751   ,  \"mm3\" -> 0.044997033026   ,  \"T\" -> 0.430000000000   ,  \"B\" -> 12.000000000000   ,  \"θ\" -> 0.000000000000   ,  \"Reoff\" -> 0.000000000000   ,  \"Imoff\" -> 0.000000000000   ,  \"στ1\" -> 0.000021533973   ,  \"στS\" -> 0.000003977444   ,  \"στN\" -> 0.000004093454   ,  \"τ11 \" -> 0.000000000000   ,  \"τ12\" -> 0.000000000000   ,  \"τ22\" -> 0.000000000000   ,  \"τN1\" -> 0.000000000000   ,  \"τN2\" -> 0.000000000000   ,  \"σηlogτ1 \" -> 0.074657261466   ,  \"σηlogτS\" -> 0.000861446772   ,  \"σηlogτN\" -> 0.050403269276   ,  \"σlogτ1\" -> 0.001884703953   ,  \"σlogτS\" -> 0.000114238081   ,  \"σlogτN\" -> 0.000953427722   ,  \"σητ1\" -> 0.000853007935   ,  \"σητS \" -> 0.000029993120   ,  \"σητN\" -> 0.000216401783    |>   , \n\"IDS0165_210310_RAW_cal__sam_\" ->   <|    \"ζ\" -> 0.031945976845   ,  \"τ1\" -> 0.019000922826   ,  \"τS\" -> 0.045624146388   ,  \"τN\" -> 0.005314716063   ,  \"τC\" -> 0.002488383471   ,  \"κ0\" -> 0.000000002954   ,  \"mm1\" -> 0.000073272643   ,  \"mm2\" -> 0.016306894362   ,  \"mm3\" -> 0.057675293464   ,  \"T\" -> 0.430000000000   ,  \"B\" -> 12.000000000000   ,  \"θ\" -> 0.000000000000   ,  \"Reoff\" -> 0.000000000000   ,  \"Imoff\" -> 0.000000000000   ,  \"στ1\" -> 0.000000000000   ,  \"στS\" -> 0.000000000000   ,  \"στN\" -> 0.000000000000   ,  \"τ11 \" -> 0.000000000000   ,  \"τ12\" -> 0.000000000000   ,  \"τ22\" -> 0.000000000000   ,  \"τN1\" -> 0.000000000000   ,  \"τN2\" -> 0.000000000000   ,  \"σηlogτ1 \" -> 0.000000000000   ,  \"σηlogτS\" -> 0.000000000000   ,  \"σηlogτN\" -> 0.000000000000   ,  \"σlogτ1\" -> 0.000000000000   ,  \"σlogτS\" -> 0.000000000000   ,  \"σlogτN\" -> 0.000000000000   ,  \"σητ1\" -> 0.000000000000   ,  \"σητS \" -> 0.000000000000   ,  \"σητN\" -> 0.000000000000    |>   , \n\"IDS0166_210310_RAW_cal__ref_\" ->   <|    \"ζ\" -> 0.024856483242   ,  \"τ1\" -> 0.010695421072   ,  \"τS\" -> 0.028584689386   ,  \"τN\" -> 0.002299338912   ,  \"τC\" -> 0.003707358018   ,  \"κ0\" -> 0.000000003388   ,  \"mm1\" -> 0.000080004626   ,  \"mm2\" -> 0.009710607688   ,  \"mm3\" -> 0.036263863406   ,  \"T\" -> 0.520000000000   ,  \"B\" -> 12.000000000000   ,  \"θ\" -> 0.000000000000   ,  \"Reoff\" -> 0.000000000000   ,  \"Imoff\" -> 0.000000000000   ,  \"στ1\" -> 0.000044725972   ,  \"στS\" -> 0.000004660348   ,  \"στN\" -> 0.000004819065   ,  \"τ11 \" -> 0.000000000000   ,  \"τ12\" -> 0.000000000000   ,  \"τ22\" -> 0.000000000000   ,  \"τN1\" -> 0.000000000000   ,  \"τN2\" -> 0.000000000000   ,  \"σηlogτ1 \" -> 0.070445110801   ,  \"σηlogτS\" -> 0.000510235434   ,  \"σηlogτN\" -> 0.049344443023   ,  \"σlogτ1\" -> 0.004181786915   ,  \"σlogτS\" -> 0.000163036495   ,  \"σlogτN\" -> 0.002095848078   ,  \"σητ1\" -> 0.000753440123   ,  \"σητS \" -> 0.000014584921   ,  \"σητN\" -> 0.000113459598    |>   , \n\"IDS0166_210310_RAW_cal__sam_\" ->   <|    \"ζ\" -> 0.023031239946   ,  \"τ1\" -> 0.018268814012   ,  \"τS\" -> 0.037269400776   ,  \"τN\" -> 0.002696792890   ,  \"τC\" -> 0.003257395394   ,  \"κ0\" -> 0.000000003720   ,  \"mm1\" -> 0.000067670174   ,  \"mm2\" -> 0.016445281937   ,  \"mm3\" -> 0.045899921957   ,  \"T\" -> 0.520000000000   ,  \"B\" -> 12.000000000000   ,  \"θ\" -> 0.000000000000   ,  \"Reoff\" -> 0.000000000000   ,  \"Imoff\" -> 0.000000000000   ,  \"στ1\" -> 0.000000000000   ,  \"στS\" -> 0.000000000000   ,  \"στN\" -> 0.000000000000   ,  \"τ11 \" -> 0.000000000000   ,  \"τ12\" -> 0.000000000000   ,  \"τ22\" -> 0.000000000000   ,  \"τN1\" -> 0.000000000000   ,  \"τN2\" -> 0.000000000000   ,  \"σηlogτ1 \" -> 0.000000000000   ,  \"σηlogτS\" -> 0.000000000000   ,  \"σηlogτN\" -> 0.000000000000   ,  \"σlogτ1\" -> 0.000000000000   ,  \"σlogτS\" -> 0.000000000000   ,  \"σlogτN\" -> 0.000000000000   ,  \"σητ1\" -> 0.000000000000   ,  \"σητS \" -> 0.000000000000   ,  \"σητN\" -> 0.000000000000    |>   , \n\"IDS0167_210310_RAW_cal__ref_\" ->   <|    \"ζ\" -> 0.023755086775   ,  \"τ1\" -> 0.012442537684   ,  \"τS\" -> 0.025226466021   ,  \"τN\" -> 0.001327754553   ,  \"τC\" -> 0.003535029288   ,  \"κ0\" -> 0.000000003992   ,  \"mm1\" -> 0.000072325961   ,  \"mm2\" -> 0.011557286901   ,  \"mm3\" -> 0.031532972498   ,  \"T\" -> 0.620000000000   ,  \"B\" -> 12.000000000000   ,  \"θ\" -> 0.000000000000   ,  \"Reoff\" -> 0.000000000000   ,  \"Imoff\" -> 0.000000000000   ,  \"στ1\" -> 0.000121120374   ,  \"στS\" -> 0.000005759367   ,  \"στN\" -> 0.000006380048   ,  \"τ11 \" -> 0.000000000000   ,  \"τ12\" -> 0.000000000000   ,  \"τ22\" -> 0.000000000000   ,  \"τN1\" -> 0.000000000000   ,  \"τN2\" -> 0.000000000000   ,  \"σηlogτ1 \" -> 0.060087437694   ,  \"σηlogτS\" -> 0.000239286620   ,  \"σηlogτN\" -> 0.047627856995   ,  \"σlogτ1\" -> 0.009734378741   ,  \"σlogτS\" -> 0.000228306534   ,  \"σlogτN\" -> 0.004805140830   ,  \"σητ1\" -> 0.000747640208   ,  \"σητS \" -> 0.000006036356   ,  \"σητN\" -> 0.000063238104    |>   , \n\"IDS0167_210310_RAW_cal__sam_\" ->   <|    \"ζ\" -> 0.019920170845   ,  \"τ1\" -> 0.016368892412   ,  \"τS\" -> 0.030579536580   ,  \"τN\" -> 0.001736017565   ,  \"τC\" -> 0.004971418152   ,  \"κ0\" -> 0.000000004410   ,  \"mm1\" -> 0.000083939556   ,  \"mm2\" -> 0.015095997595   ,  \"mm3\" -> 0.039119658918   ,  \"T\" -> 0.620000000000   ,  \"B\" -> 12.000000000000   ,  \"θ\" ->
